vi "标样核查配置.vi"() -> (2 "确认输出":bool)   [LabVIEW 2016, in "斯坦道多参数.lvlib"]
panel:
  in  "藻密度标样值":dbl caption="藻密度"
  in  "叶绿素a标样值":dbl caption="叶绿素a"
  in  "藻密度启用":bool
  in  "叶绿素a启用":bool
  in  "保存组数":dbl=1.0
  in  "浊度启用":bool
  in  "电导率启用":bool
  in  "溶解氧启用":bool
  in  "pH启用":bool
  in  "浊度标样值":dbl caption="浊度"
  in  "电导率标样值":dbl caption="电导率"
  in  "溶解氧标样值":dbl caption="溶解氧"
  in  "pH标样值":dbl caption="pH"
  in  "取消":bool
  in  "确定":bool
  in  "数据保存间隔":dbl=1.0
  # "请输入数据保存间隔"
  # "保存组数"
  # "min"
  # "组"
  # "请选择启动项"
  # "请输入各参数标样值"
  # "mg/L"
  # "μS/cm"
  # "NTU"
  # "μg/L"
  # "cells/mL"
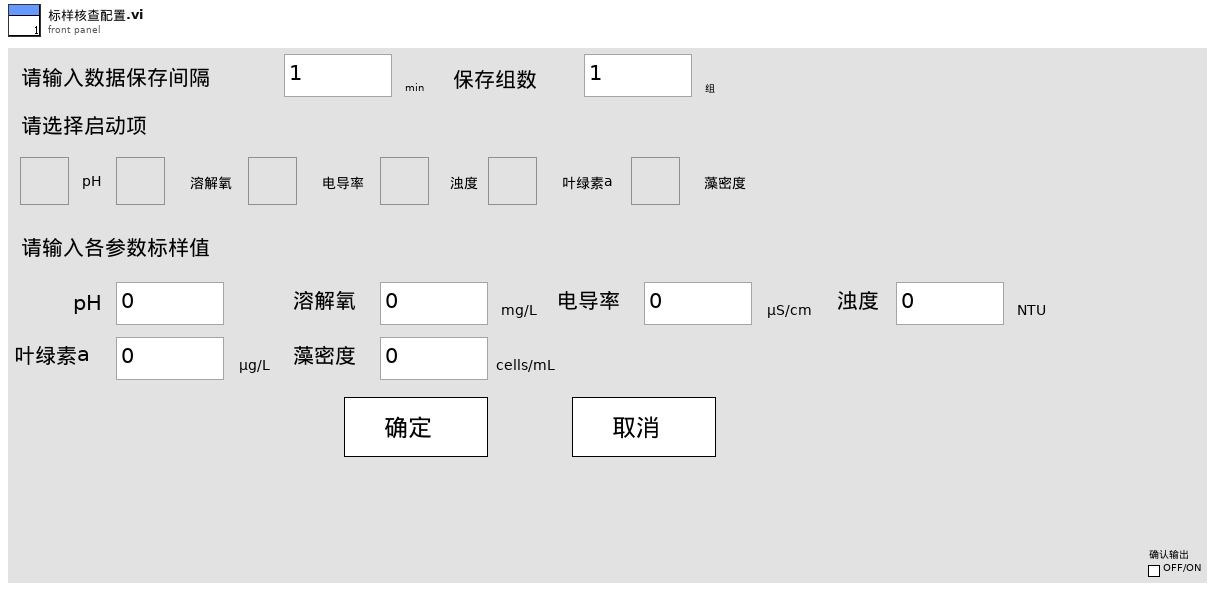
[diagram p1: front panel]
types:
  T1 = cluster{"数据保存间隔":dbl, "保存组数":dbl, "水温标样值":dbl, "pH标样值":dbl, "溶解氧标样值":dbl, "电导率标样值":dbl, "浊度标样值":dbl, "叶绿素a标样值":dbl, "藻密度标样值":dbl, "pH启用":bool, "溶解氧启用":bool, "电导率启用":bool, "浊度启用":bool, "叶绿素a启用":bool, "藻密度启用":bool}
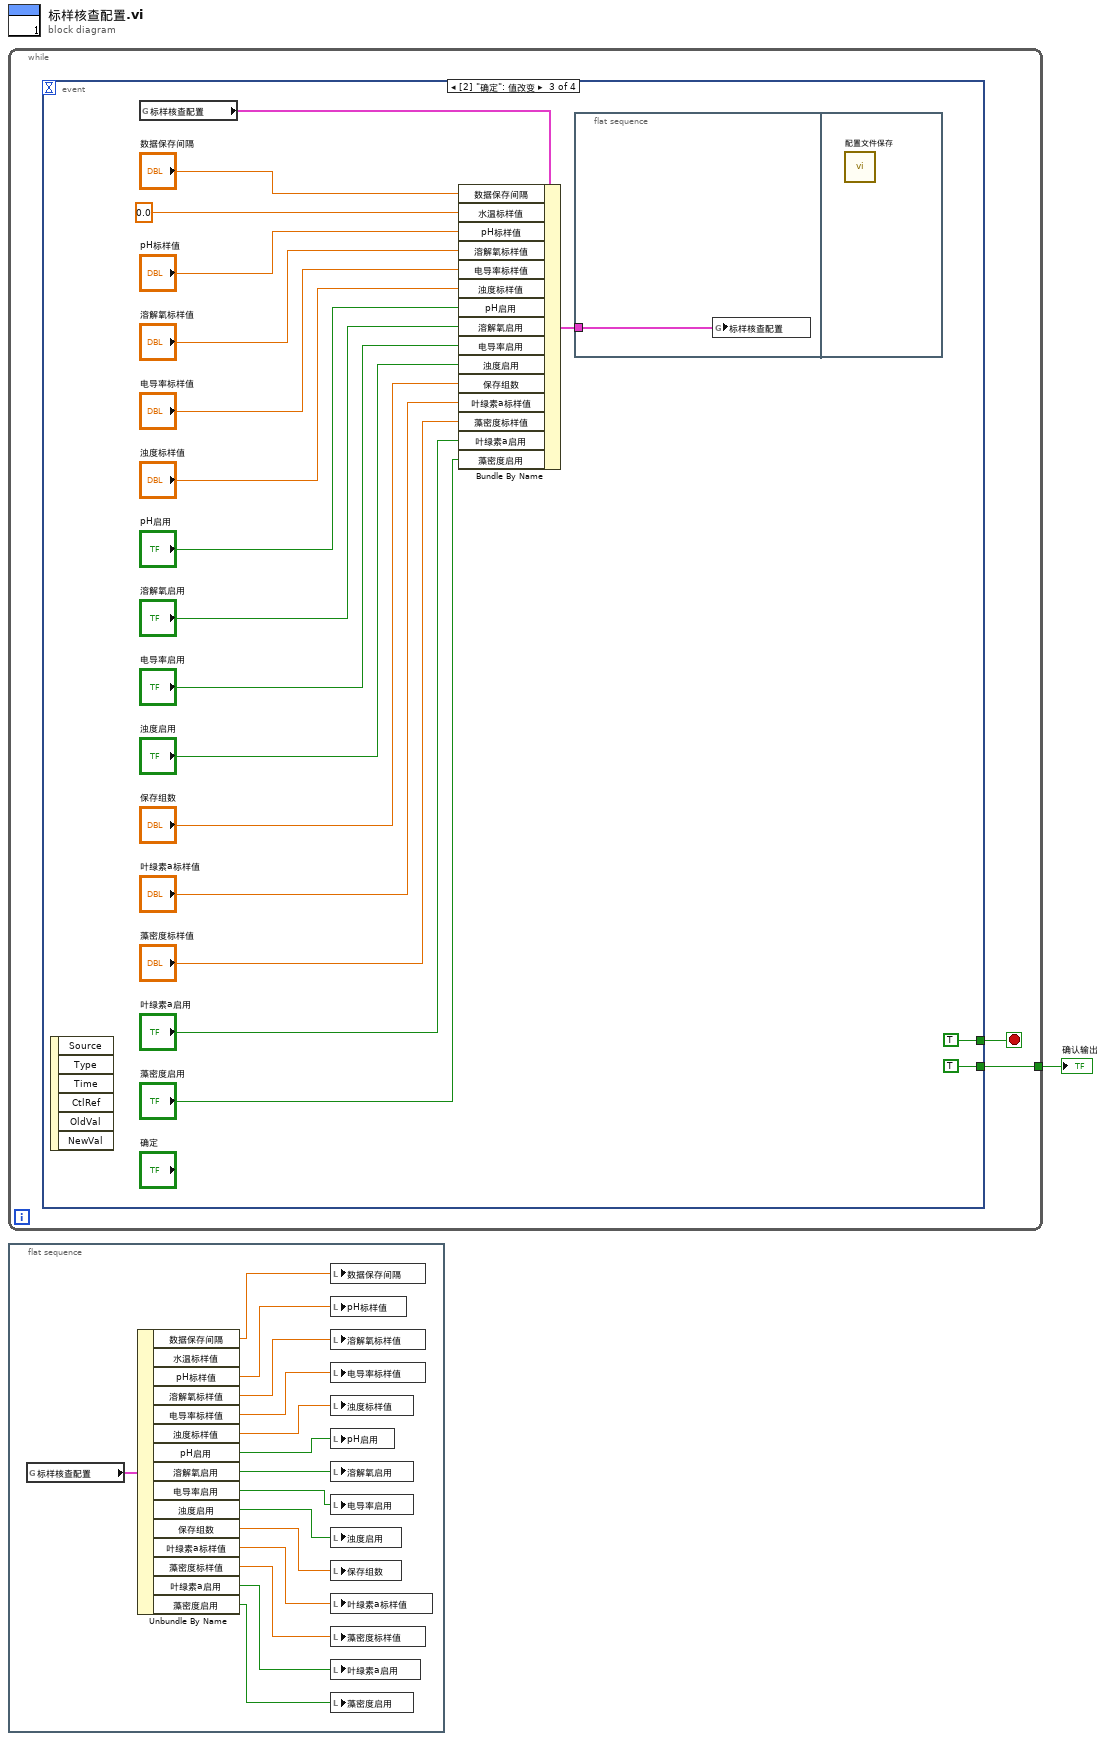
[diagram p0: block diagram]
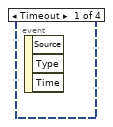
[diagram p2: hidden frame]
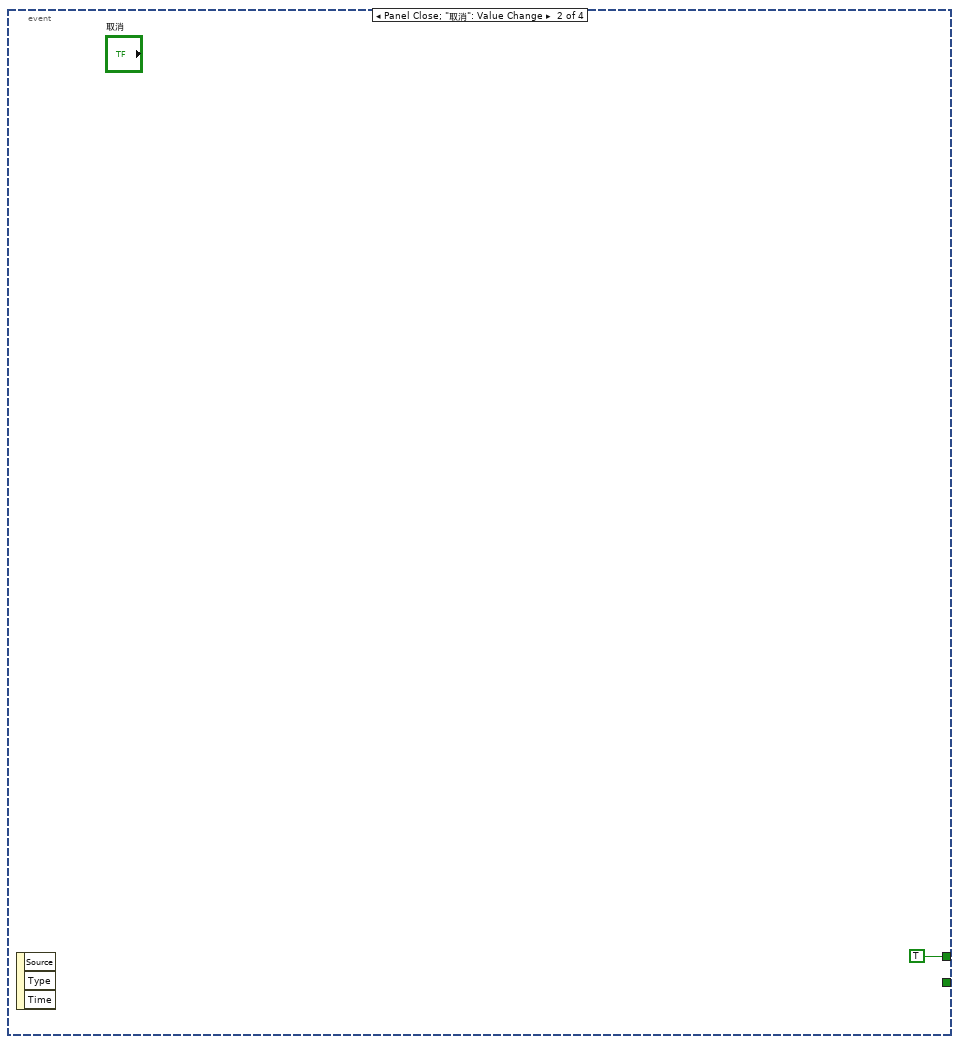
[diagram p3: hidden frame]
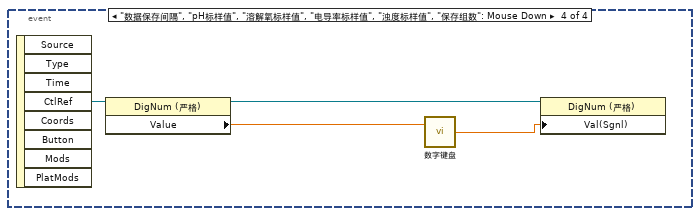
[diagram p4: hidden frame]
diagram:
  n1 = while {
    tunnel: [w2] -> w1
    stop <- w3 stop-if-true
    n2 = event shown="[2] \"确定\": 值改变" {
      selector: _ -> [_ _ _ _]
      dyn-events: _ -> [_ _ _ _]
      timeout: _ -> [_ _ _ _]
      tunnel: [_ TRUE TRUE _] -> w3
      tunnel: [_ _ TRUE _] -> w2
      event Timeout {
        n3 = event-data() -> ()  [unwired: 1 in, 3 out]
      }
      event Panel Close; "取消": Value Change {
        n4 = event-data() -> ()  [unwired: 1 in, 3 out]
      }
      event "确定": Value Change {
        n5 = event-data() -> ()  [unwired: 1 in, 6 out]
        n6 = global read "断电保存变量.vi" "标样核查配置"() -> (w22:T1)
        n7 = Bundle By Name(cluster=w22, "数据保存间隔"="数据保存间隔", "水温标样值"=0.0, "pH标样值"="pH标样值", "溶解氧标样值"="溶解氧标样值", "电导率标样值"="电导率标样值", "浊度标样值"="浊度标样值", "pH启用"="pH启用", "溶解氧启用"="溶解氧启用", "电导率启用"="电导率启用", "浊度启用"="浊度启用", "保存组数"="保存组数", "叶绿素a标样值"="叶绿素a标样值", "藻密度标样值"="藻密度标样值", "叶绿素a启用"="叶绿素a启用", "藻密度启用"="藻密度启用") -> (w21:T1)
        n8 = flat-sequence {
          tunnel: w21 -> [w24]
          frame #0 {
            n9 = global write "断电保存变量.vi" "标样核查配置"(w24) -> ()
          }
          frame #1 {
            n10 = call "配置文件保存.vi"() -> ()  [unwired: 12 in]
          }
        }
      }
      event "数据保存间隔", "pH标样值", "溶解氧标样值", "电导率标样值", "浊度标样值", "保存组数": Mouse Down {
        n11 = event-data() -> ("CtlRef"=w28:refnum<vi>)  [unwired: 1 in, 7 out]
        n12 = property class="DigNum (严格)"(reference=w28) -> (reference out=w25:refnum<vi>, "Value"=w27:dbl)  [unwired: 1 in, 1 out]
        n13 = call "数字键盘.vi"("OldNumber"=w27) -> ("NewNumber"=w26:dbl)  [unwired: 1 in]
        n14 = property class="DigNum (严格)"(reference=w25, "Val(Sgnl)"=w26) -> ()  [unwired: 1 in, 2 out]
      }
    }
  }
  "确认输出" <- w1
  n15 = flat-sequence {
    frame #0 {
      n16 = global read "断电保存变量.vi" "标样核查配置"() -> (w43:T1)
      n17 = Unbundle By Name(w43) -> ("数据保存间隔"=w42:dbl, "pH标样值"=w38:dbl, "溶解氧标样值"=w39:dbl, "电导率标样值"=w40:dbl, "浊度标样值"=w41:dbl, "pH启用"=w37:bool, "溶解氧启用"=w36:bool, "电导率启用"=w35:bool, "浊度启用"=w34:bool, "保存组数"=w33:dbl, "叶绿素a标样值"=w32:dbl, "藻密度标样值"=w31:dbl, "叶绿素a启用"=w30:bool, "藻密度启用"=w29:bool)  [unwired: 1 out]
      n18 = local write "数据保存间隔"(w42) -> ()
      n19 = local write "pH标样值"(w38) -> ()
      n20 = local write "溶解氧标样值"(w39) -> ()
      n21 = local write "电导率标样值"(w40) -> ()
      n22 = local write "浊度标样值"(w41) -> ()
      n23 = local write "pH启用"(w37) -> ()
      n24 = local write "溶解氧启用"(w36) -> ()
      n25 = local write "电导率启用"(w35) -> ()
      n26 = local write "浊度启用"(w34) -> ()
      n27 = local write "保存组数"(w33) -> ()
      n28 = local write "叶绿素a标样值"(w32) -> ()
      n29 = local write "藻密度标样值"(w31) -> ()
      n30 = local write "叶绿素a启用"(w30) -> ()
      n31 = local write "藻密度启用"(w29) -> ()
    }
  }
